vi "Wait on Stop Sync.vi"(8 "error in (no error)":errorcluster, 10 "Wait for Module to stop?":bool=TRUE, 11 "Module ID":i32) -> (0 "error out":errorcluster)   [LabVIEW 2020, in "My Cloneable Module.lvlib"]
doc: "Wait on the rendezvous that synchronizes the request to stop the module and the module stopping.\n\n_____\nBased on Delacor QMH Project Template 5.0.0.82."
uses:
  My Cloneable Module.lvlib
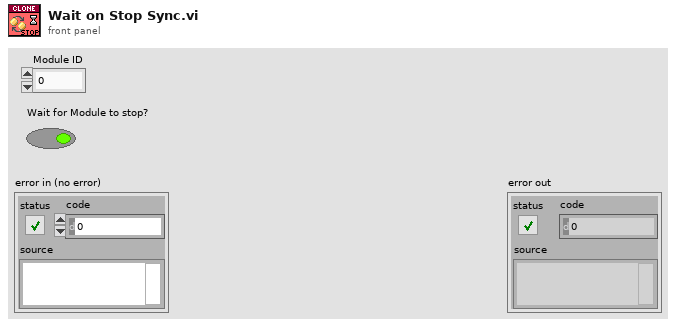
[diagram p1: front panel]
types:
  T1 = typedef "My Cloneable Module.lvlib/Broadcast Events--cluster.ctl" = cluster{"Module Did Init":refnum<user-event>, "Status Updated":refnum<user-event>, "Error Reported":refnum<user-event>, "Did Something":refnum<user-event>, "Module Did Stop":refnum<user-event>, "Update Module Execution Status":refnum<user-event>}
  T2 = typedef "Rendezvous RefNum" = refnum<k1>
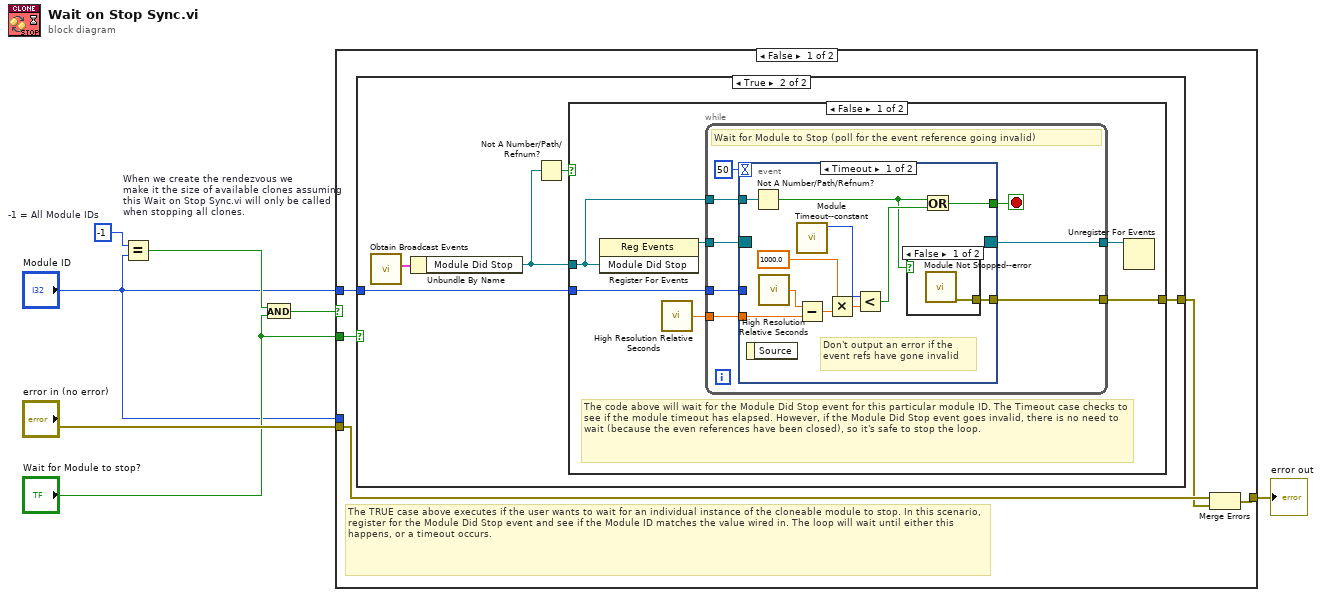
[diagram p0: block diagram]
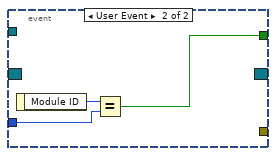
[diagram p4: hidden frame]
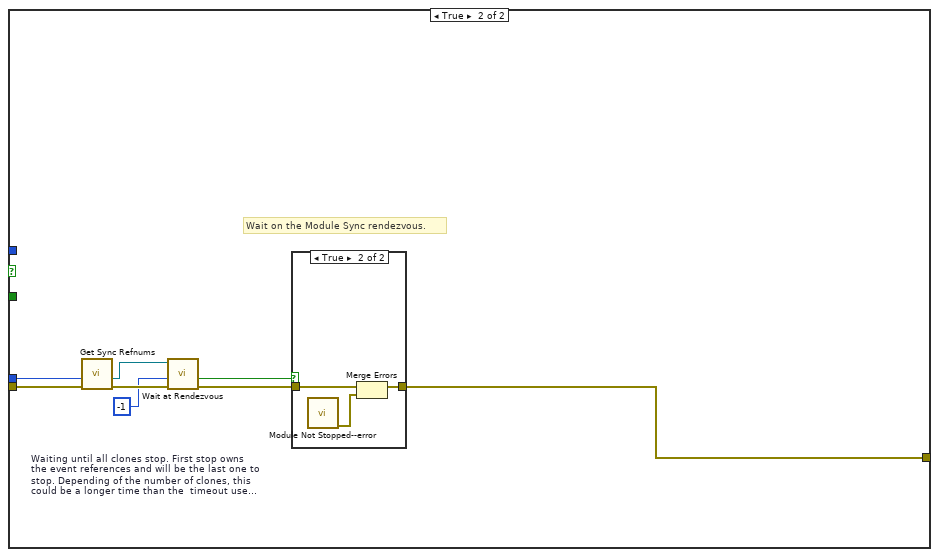
[diagram p6: hidden frame]
diagram:
  w5 = -1  # -1 = All Module IDs
  n1 = Equal? "When we create the rendezvous we\nmake it the size of available clones assuming this Wait on Stop Sync.vi will only be called when stopping all clones."(x=w5, y="Module ID") -> (x = y?=w4:bool)
  n2 = And(x=w4, y="Wait for Module to stop?") -> (x .and. y?=w3:bool)
  n3 = case shown="False" w3 {
    tunnel: "error in (no error)" -> [w12 w54]
    tunnel: [w9 w49] -> w6
    tunnel: "Module ID" -> [_ w48]
    tunnel: "Wait for Module to stop?" -> [w11 _]
    tunnel: "Module ID" -> [w10 _]
    frame False {
      # "The TRUE case above executes if the user wants to wait for an individual instance of the cloneable module to stop. In this scenario, register for the Module Did Stop event and see if the Module ID matches the value wired in. The loop will wait until either this happens, or a timeout occurs."
      n4 = case shown="True" w11 {
        tunnel: w10 -> [_ w16]
        tunnel: [_ w15] -> w8
        frame False {
          # "User does not want to wait for the module to stop."
        }
        frame True {
          n5 = call "Obtain Broadcast Events.vi"() -> ("My Cloneable Module Broadcast Events"=w17:T1)  [unwired: 10 in, 1 out]
          n6 = Unbundle By Name(w17) -> ("Module Did Stop"=w14:refnum<user-event>)
          n7 = Not A Number/Path/Refnum?(number/path/refnum=w14) -> (NaN/Path/Refnum?=w13:bool)
          n8 = case shown="False" w13 {
            tunnel: w16 -> [w22 _]
            tunnel: [w21 _] -> w15
            tunnel: w14 -> [w19 _]
            frame False {
              # "The code above will wait for the Module Did Stop event for this particular module ID. The Timeout case checks to see if the module timeout has elapsed. However, if the Module Did Stop event goes invalid, there is no need to wait (because the even references have been closed), so it's safe to stop the loop."
              n9 = register-events(w19) -> (reference out=w23:refnum<event-registration>)  [unwired: 2 in, 1 out]
              n10 = call <vilib>:"High Resolution Relative Seconds.vi"() -> ("relative seconds"=w18:dbl)
              n11 = while {
                tunnel: w23 -> [w31]
                tunnel: w22 -> [w29]
                tunnel: [w28] -> w21
                tunnel: [w27] -> w20
                tunnel: w19 -> [w25]
                tunnel: w18 -> [w24]
                stop <- w30 stop-if-true
                # "Wait for Module to Stop (poll for the event reference going invalid)"
                n12 = event shown="[0] Timeout" {
                  selector: w31 -> [_ _]
                  dyn-events: [_ _] -> w27
                  timeout: 50 -> [_ _]
                  tunnel: [w40 w44] -> w30
                  tunnel: w29 -> [_ w45]
                  tunnel: [w42 _] -> w28
                  tunnel: w25 -> [w41 _]
                  tunnel: w24 -> [w39 _]
                  event Timeout {
                    # "Don't output an error if the event refs have gone invalid"
                    n13 = event-data() -> ()  [unwired: 1 in, 1 out]
                    n14 = Not A Number/Path/Refnum?(number/path/refnum=w41) -> (NaN/Path/Refnum?=w32:bool)
                    n15 = call <vilib>:"High Resolution Relative Seconds.vi"() -> ("relative seconds"=w38:dbl)
                    n16 = call "Module Timeout--constant.vi"() -> ("Module Timeout"=w34:i32)  [unwired: 11 in]
                    n17 = Subtract(x=w38, y=w39) -> (x-y=w37:dbl)
                    n18 = Multiply(x=1000.0, y=w37) -> (x*y=w35:dbl)
                    n19 = Less?(x=w34, y=w35) -> (x < y?=w33:bool)
                    n20 = case shown="False" w32 {
                      tunnel: [w43 _] -> w42
                      frame False {
                        n21 = call "Module Not Stopped--error.vi"() -> ("error out"=w43:errorcluster)  [unwired: 11 in]
                      }
                      frame True {
                      }
                    }
                    n22 = Or(x=w32, y=w33) -> (x .or. y?=w40:bool)
                  }
                  event User Event {
                    n23 = event-data() -> ("Module ID"=w46:i32)  [unwired: 1 in]
                    n24 = Equal?(x=w46, y=w45) -> (x = y?=w44:bool)
                  }
                }
              }
              n25 = Unregister For Events(event registration refnum=w20) -> ()  [unwired: 1 in, 1 out]
            }
            frame True {
              # "Don't wait if the Module Did Stop reference has already been closed"
            }
          }
        }
      }
      n26 = Merge Errors(w12, w8) -> (w9:errorcluster)
    }
    frame True {
      w52 = -1  # Waiting until all clones stop. First stop owns the event references and will be the last one to stop. Depending of the number of clones, this could be a longer time than the  timeout used for the other rendezvous.
      # "Wait on the Module Sync rendezvous."
      n27 = call "Get Sync Refnums.vi"("error in (no error)"=w54, "Module ID"=w48) -> ("error out"=w53:errorcluster, "Stop Sync"=w47:T2)  [unwired: 6 in, 2 out]
      n28 = call <vilib>:"Wait at Rendezvous.vi"("error in (no error)"=w53, "ms timeout (-1)"=w52, "rendezvous"=w47) -> ("error out"=w51:errorcluster, "timed out"=w50:bool)  [unwired: 2 in, 1 out]
      n29 = case shown="True" w50 {
        tunnel: w51 -> [w55 w58]
        tunnel: [w55 w57] -> w49
        frame False {
        }
        frame True {
          n30 = call "Module Not Stopped--error.vi"() -> ("error out"=w56:errorcluster)  [unwired: 11 in]
          n31 = Merge Errors(w58, w56) -> (w57:errorcluster)
        }
      }
    }
  }
  "error out" <- w6
